vi "wash sample loop.vi"   [LabVIEW 2023]
types:
  T1 = enum16{"Initialize", "Absolute Position", "Relative Pickup", "Relative Dispense", "Swich valve", "Bypass"}
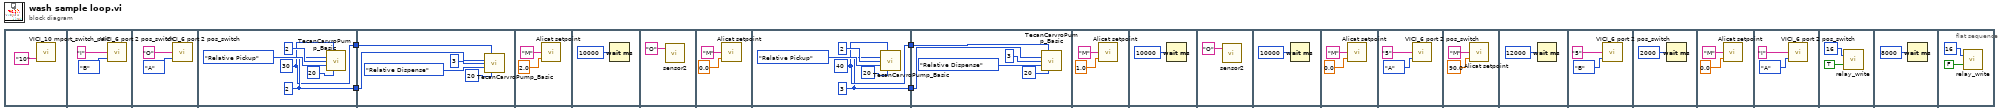
[diagram p0: block diagram]
diagram:
  n1 = flat-sequence {
    tunnel: [w11] -> w4
    tunnel: [w10] -> w3
    tunnel: w4 -> [w16]
    tunnel: w3 -> [w15]
    tunnel: [w27] -> w2
    tunnel: [w26] -> w1
    tunnel: w2 -> [w32]
    tunnel: w1 -> [w31]
    frame #0 {
      n2 = call "VICI_10 mport_switch_pair.vi"("Go to position"="10") -> ()  [unwired: 3 in, 1 out]
    }
    frame #1 {
      n3 = call "VICI_6 port 2 pos_switch.vi"("Switch to position (A/B)"=enum16{"A", "B"}."B", "Valve ID"="I") -> ()  [unwired: 2 in, 1 out]
    }
    frame #2 {
      n4 = call "VICI_6 port 2 pos_switch.vi"("Switch to position (A/B)"=enum16{"A", "B"}."A", "Valve ID"="O") -> ()  [unwired: 2 in, 1 out]
    }
    frame #3 {
      w11 = u8 2 ("TecanPump address")
      w10 = u16 30 ("Volume (μL)")
      n5 = call "TecanCarvroPump_Basic.vi"("Volume (μL)"=w10, "TecanPump address"=w11, "Valve"=u8 2, "Mode"=T1."Relative Pickup", "Speed (μL/s)"=u16 20) -> ()  [unwired: 10 in, 1 out]
    }
    frame #4 {
      n6 = call "TecanCarvroPump_Basic.vi"("Volume (μL)"=w15, "TecanPump address"=w16, "Valve"=u8 3, "Mode"=T1."Relative Dispense", "Speed (μL/s)"=u16 20) -> ()  [unwired: 10 in, 1 out]
    }
    frame #5 {
      n7 = call "Alicat setpoint.vi"("Setpoint"=2.0, "Unit ID"="M") -> ()  [unwired: 3 in]
    }
    frame #6 {
      n8 = Wait (ms)(milliseconds to wait=u32 10000) -> ()  [unwired: 1 out]
    }
    frame #7 {
      n9 = call "sensor2.vi"("Sensor"="O") -> ()  [unwired: 1 in, 2 out]
    }
    frame #8 {
      n10 = call "Alicat setpoint.vi"("Setpoint"=0.0, "Unit ID"="M") -> ()  [unwired: 3 in]
    }
    frame #9 {
      w26 = u8 3 ("TecanPump address")
      w27 = u16 40 ("Volume (μL)")
      n11 = call "TecanCarvroPump_Basic.vi"("Volume (μL)"=w27, "TecanPump address"=w26, "Valve"=u8 2, "Mode"=T1."Relative Pickup", "Speed (μL/s)"=u16 20) -> ()  [unwired: 10 in, 1 out]
    }
    frame #10 {
      n12 = call "TecanCarvroPump_Basic.vi"("Volume (μL)"=w32, "TecanPump address"=w31, "Valve"=u8 3, "Mode"=T1."Relative Dispense", "Speed (μL/s)"=u16 20) -> ()  [unwired: 10 in, 1 out]
    }
    frame #11 {
      n13 = call "Alicat setpoint.vi"("Setpoint"=1.0, "Unit ID"="M") -> ()  [unwired: 3 in]
    }
    frame #12 {
      n14 = Wait (ms)(milliseconds to wait=u32 10000) -> ()  [unwired: 1 out]
    }
    frame #13 {
      n15 = call "sensor2.vi"("Sensor"="O") -> ()  [unwired: 1 in, 2 out]
    }
    frame #14 {
      n16 = Wait (ms)(milliseconds to wait=u32 10000) -> ()  [unwired: 1 out]
    }
    frame #15 {
      n17 = call "Alicat setpoint.vi"("Setpoint"=0.0, "Unit ID"="M") -> ()  [unwired: 3 in]
    }
    frame #16 {
      n18 = call "VICI_6 port 2 pos_switch.vi"("Switch to position (A/B)"=enum16{"A", "B"}."A", "Valve ID"="5") -> ()  [unwired: 2 in, 1 out]
    }
    frame #17 {
      n19 = call "Alicat setpoint.vi"("Setpoint"=90.0, "Unit ID"="M") -> ()  [unwired: 3 in]
    }
    frame #18 {
      n20 = Wait (ms)(milliseconds to wait=u32 12000) -> ()  [unwired: 1 out]
    }
    frame #19 {
      n21 = call "VICI_6 port 2 pos_switch.vi"("Switch to position (A/B)"=enum16{"A", "B"}."B", "Valve ID"="5") -> ()  [unwired: 2 in, 1 out]
    }
    frame #20 {
      n22 = Wait (ms)(milliseconds to wait=u32 2000) -> ()  [unwired: 1 out]
    }
    frame #21 {
      n23 = call "Alicat setpoint.vi"("Setpoint"=0.0, "Unit ID"="M") -> ()  [unwired: 3 in]
    }
    frame #22 {
      n24 = call "VICI_6 port 2 pos_switch.vi"("Switch to position (A/B)"=enum16{"A", "B"}."A", "Valve ID"="I") -> ()  [unwired: 2 in, 1 out]
    }
    frame #23 {
      n25 = call "relay_write.vi"("on/off"=TRUE, "No."=u8 16) -> ()  [unwired: 1 out]
    }
    frame #24 {
      n26 = Wait (ms)(milliseconds to wait=u32 8000) -> ()  [unwired: 1 out]
    }
    frame #25 {
      n27 = call "relay_write.vi"("on/off"=FALSE, "No."=u8 16) -> ()  [unwired: 1 out]
    }
  }
